vi "EMG_DESC_main_v003.vi"() -> ()   [LabVIEW 2019]
uses:
  <vilib>/Utility/file.llb/Read Delimited Spreadsheet (DBL).vi
  <vilib>/Utility/file.llb/Read Delimited Spreadsheet (string).vi
panel:
  out "Waveform Graph 3":dbl[](graph)
  in  "Lowpass (High) cutoff freq":dbl=200.0
  out "Waveform Graph 2":dbl[](graph)
  out "Waveform Graph":dbl[](graph)
  in  "Highpass (Low) cutoff freq":dbl=20.0 format="%0.4f"
  in  "Raw Threshold":dbl
  out "Thresholded Enveloped Signal Graph":dbl[](graph)
  out "Thresholded Raw Signal Graph":dbl[][](graph)
  in  "Envelopped Threshold":dbl
  out "Enveloped signal Graph":waveform(dbl)(graph)
  in  "Desired Signal":enum16{"Raw", "Env"}(ring)
  out "Impoting Path":path
  out "Raw signal Graph":waveform(dbl)(graph)
  in  "Samping Frequency":dbl=2000.0
  out "Headers":string[](array[string])
  out "Data":dbl[][](array[numeric])
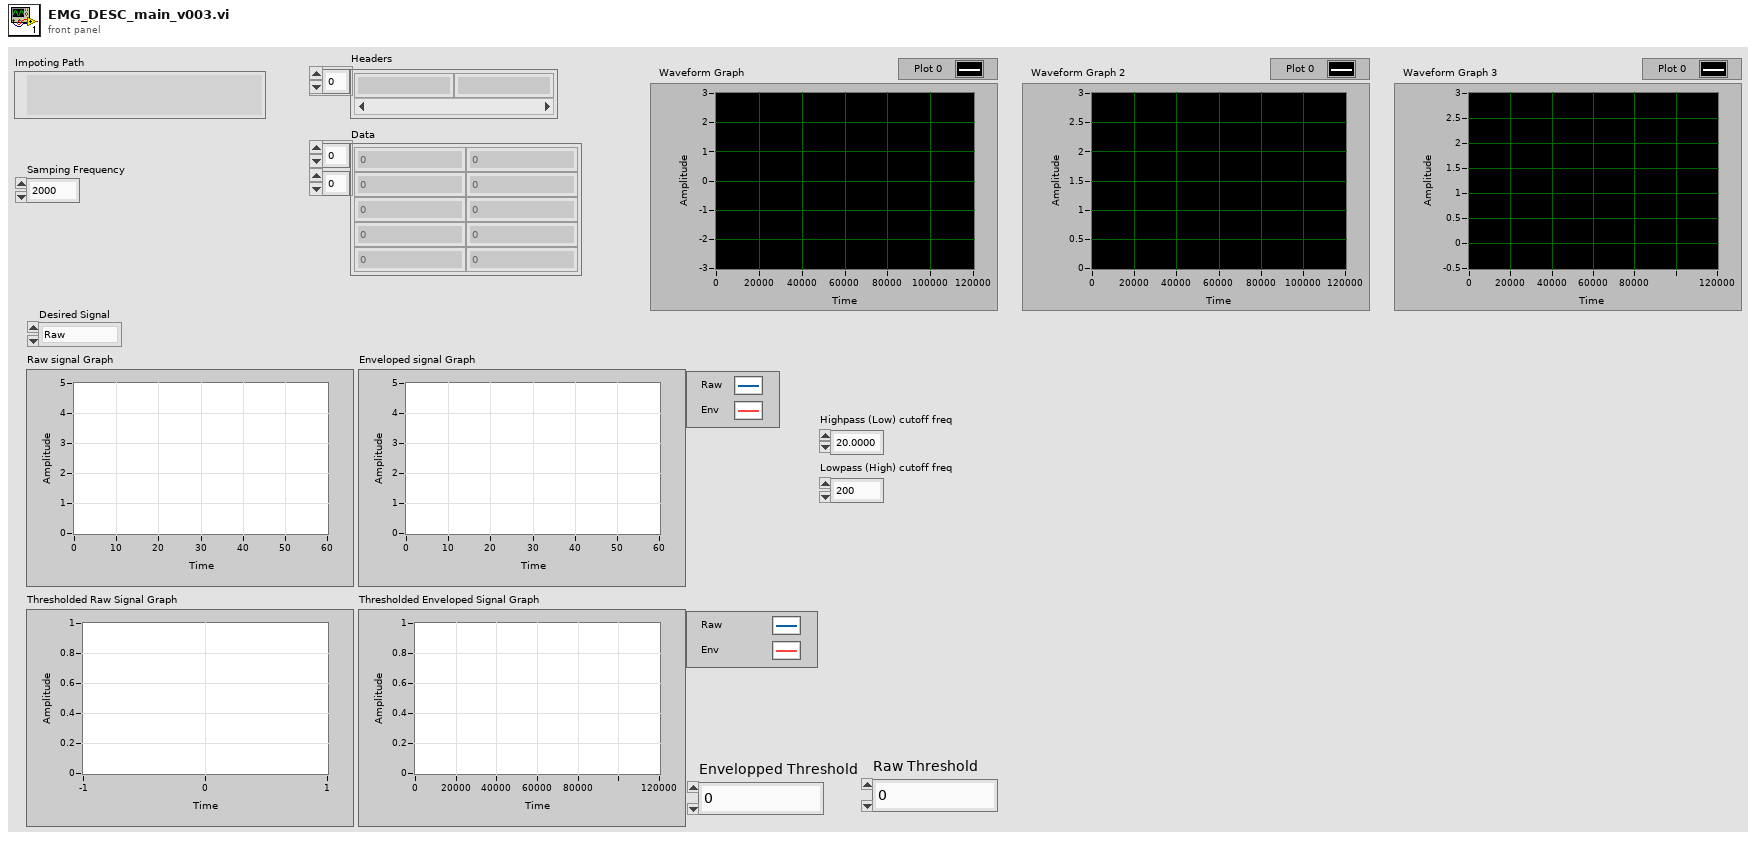
[diagram p1: front panel]
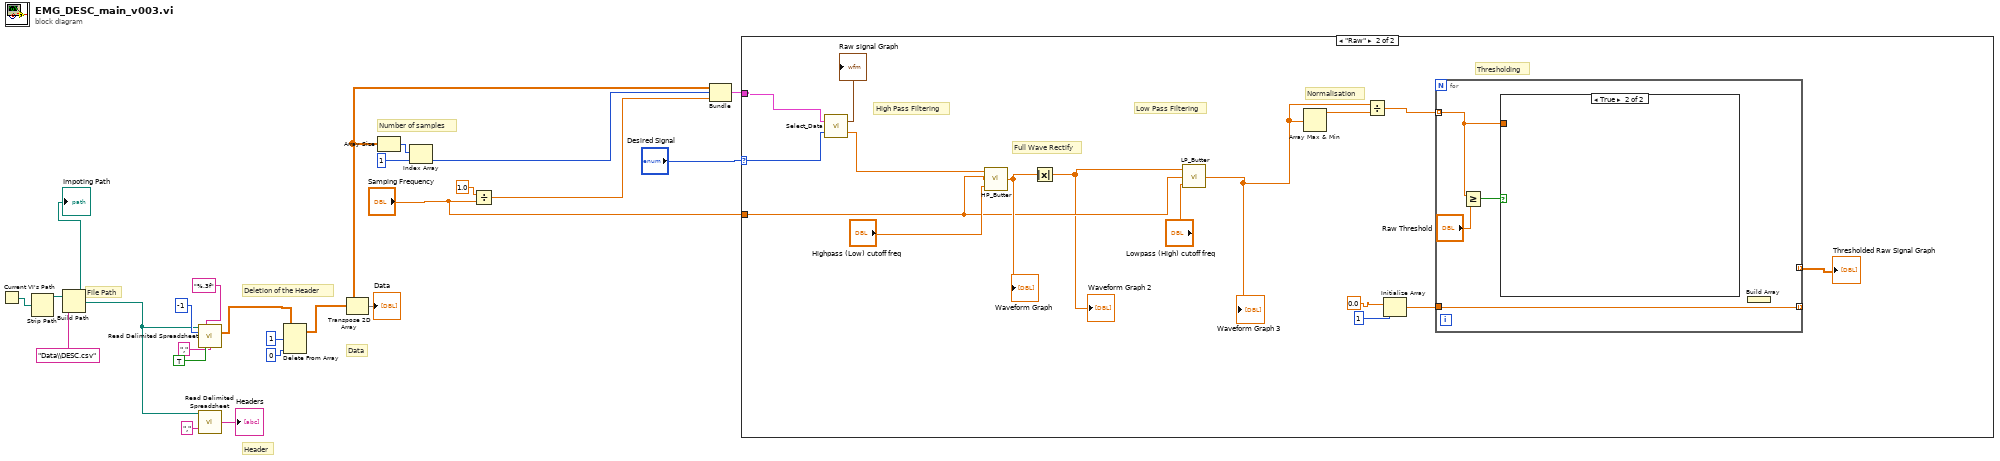
[diagram p0: block diagram]
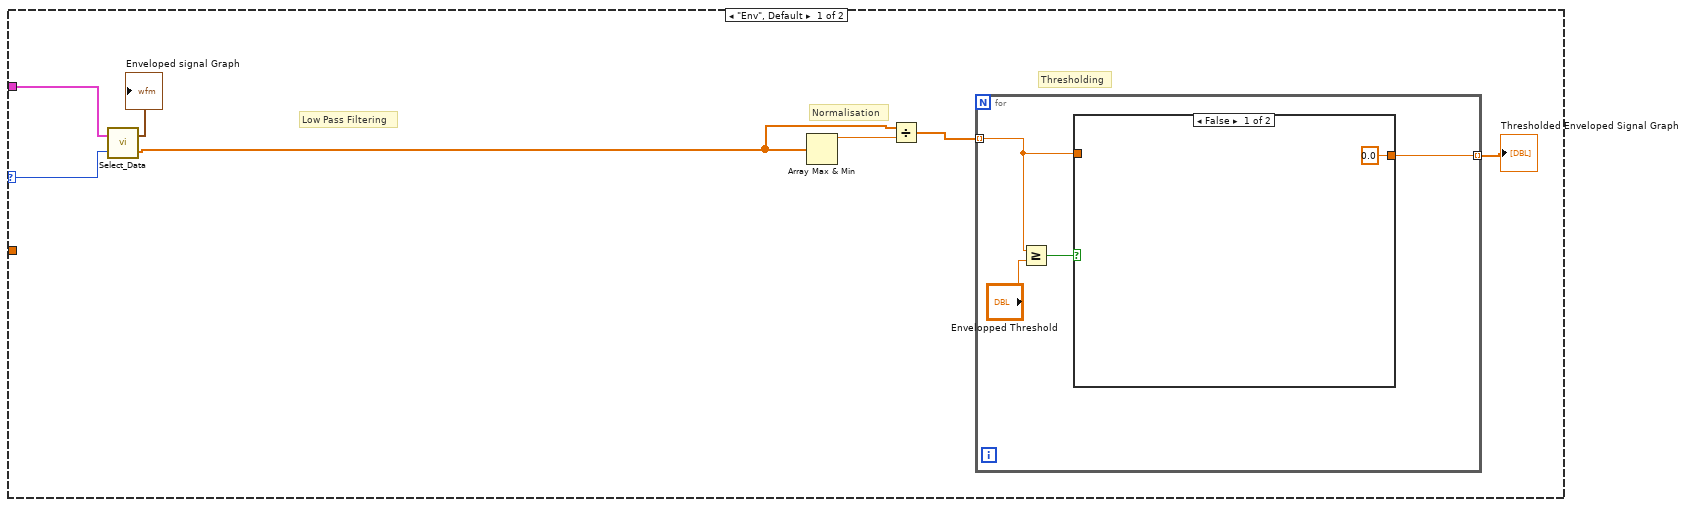
[diagram p2: hidden frame]
diagram:
  # "Header"
  # "Data"
  # "Deletion of the Header"
  # "File Path"
  # "Number of samples"
  n1 = Current VI's Path() -> (path=w11:path)
  n2 = Strip Path(path=w11) -> (stripped path=w10:path)  [unwired: 1 out]
  n3 = Build Path(base path=w10, name or relative path="Data\\DESC.csv") -> (appended path=w9:path)
  "Impoting Path" <- w9
  n4 = call-poly <vilib>:"Read Delimited Spreadsheet.vi"("file path (dialog if empty)"=w9, "format (%.3f)"="%.3f", "number of rows (all:-1)"=-1, "transpose? (F)"=TRUE, "delimiter (\\t)"="," ("delimiter (\\t)")) -> ("all rows"=w16:dbl[][])  [unwired: 5 in, 5 out]
  n5 = call-poly <vilib>:"Read Delimited Spreadsheet.vi"("file path (dialog if empty)"=w9, "delimiter (\\t)"="," ("delimiter (\\t)")) -> ("first row"=→"Headers":string[])  [unwired: 8 in, 5 out]
  n6 = Delete From Array(array=w16, length=1 ("index"), index (col)=0 ("index")) -> (array with subset deleted=w6:dbl[][])  [unwired: 1 in, 1 out]
  n7 = Transpose 2D Array(2D array=w6) -> (transposed array=→"Data":dbl[][])
  n8 = Array Size(array=w6) -> (size(s)=w14:i32[])
  n9 = Index Array(array=w14, index=1) -> (element=w5:i32)
  n10 = Divide(x=1.0, y="Samping Frequency") -> (x/y=w1:dbl)
  n11 = Bundle("all rows"=w6, w5, w1) -> (w4:cluster{"all rows":dbl[][], i32, dbl})  [unwired: 1 in]
  n12 = case shown="\"Raw\"" "Desired Signal" {
    selector: "Desired Signal" -> [w25 w49]
    tunnel: w4 -> [w26 w50]
    tunnel: "Samping Frequency" -> [_ w44]
    frame "Env", Default {
      # "Low Pass Filtering"
      # "Thresholding"
      # "Normalisation"
      n13 = call "Select_Data.vi"("Desired Signal"=w25, "Cluster"=w26) -> ("Signal Sequence"=w24:dbl[], "Waveform"=→"Enveloped signal Graph":waveform(dbl))
      n14 = Array Max & Min(array=w24) -> (max value=w30:dbl)  [unwired: 3 out]
      n15 = Divide(x=w24, y=w30) -> (x/y=w29:dbl[])
      n16 = for {
        tunnel: w29 -> [w33] mode=indexing
        tunnel: [w32] -> w28 mode=indexing
        n17 = Greater Or Equal?(x=w33, y="Envelopped Threshold") -> (x >= y?=w34:bool)
        n18 = case shown="False" w34 {
          tunnel: [0.0 ("Numeric") w36] -> w32
          tunnel: w33 -> [_ w36]
          frame False {
          }
          frame True {
          }
        }
      }
      "Thresholded Enveloped Signal Graph" <- w28
    }
    frame "Raw" {
      # "Full Wave Rectify"
      # "High Pass Filtering"
      # "Low Pass Filtering"
      # "Thresholding"
      # "Normalisation"
      n19 = call "Select_Data.vi"("Desired Signal"=w49, "Cluster"=w50) -> ("Signal Sequence"=w47:dbl[], "Waveform"=→"Raw signal Graph":waveform(dbl))
      n20 = call "HP_Butter.vi"("low cutoff freq: fl"="Highpass (Low) cutoff freq", "Samping Frequency"=w44, "Signal Sequence"=w47) -> ("Array"=w45:dbl[])
      "Waveform Graph" <- w45
      n21 = Absolute Value(x=w45) -> (abs(x)=w43:dbl[])
      "Waveform Graph 2" <- w43
      n22 = call "LP_Butter.vi"("High cutoff freq"="Lowpass (High) cutoff freq", "Samping Frequency"=w44, "Signal Sequence"=w43) -> ("reversed array"=w41:dbl[])
      "Waveform Graph 3" <- w41
      n23 = Array Max & Min(array=w41) -> (max value=w52:dbl)  [unwired: 3 out]
      n24 = Divide(x=w41, y=w52) -> (x/y=w51:dbl[])
      n25 = Initialize Array(0.0 ("element"), 1 ("dimension size")) -> (w37:dbl[])
      n26 = for {
        tunnel: w51 -> [w56] mode=indexing
        tunnel: [w54] -> w40 mode=indexing
        tunnel: w37 -> [w53]
        tunnel: [w53] -> _ mode=indexing
        n27 = Greater Or Equal?(x=w56, y="Raw Threshold") -> (x >= y?=w57:bool)
        n28 = case shown="True" w57 {
          tunnel: w56 -> [_ w58]
          frame False {
          }
          frame True {
          }
        }
        n29 = Build Array() -> ()  [unwired: 1 in, 1 out]
      }
      "Thresholded Raw Signal Graph" <- w40
    }
  }
